vi "Set BufferLastReadsDBL.vi"(10 "BufferLastReadings DBL":refnum<class "BufferLastReadsDBL.lvclass">, 11 "AI DAQmx Cont CFG in":refnum<class "AI DAQmx Cont CFG.lvclass">) -> (3 "AI DAQmx Cont CFG out":refnum<class "AI DAQmx Cont CFG.lvclass">)   [LabVIEW 2023, in "AI DAQmx Cont CFG.lvclass"]
uses:
  AI DAQmx Cont CFG.lvclass
  DAQmx/BufferLastReadingsDBL/BufferLastReadsDBL.lvclass
  AI DAQmx Cont CFG.lvclass/AI DAQmx Cont CFG.ctl
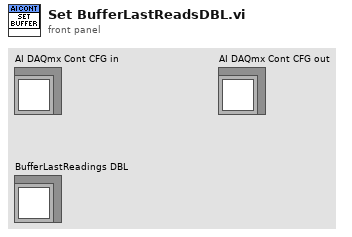
[diagram p1: front panel]
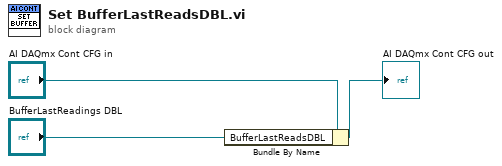
[diagram p0: block diagram]
diagram:
  n1 = Bundle By Name(cluster="AI DAQmx Cont CFG in", "BufferLastReadsDBL"="BufferLastReadings DBL") -> (→"AI DAQmx Cont CFG out":refnum<class "AI DAQmx Cont CFG.lvclass">)
